vi "saveData.vi"(1 "display write dialog?":bool, 2 "append to file?":bool, 3 "Block Timing":T1) -> (0 "error out":errorcluster)   [LabVIEW 2013]
uses:
  Controls/blockTiming.ctl
  Globals/measurementGlobal.vi
panel:
  out "File Status":string="File not appended"
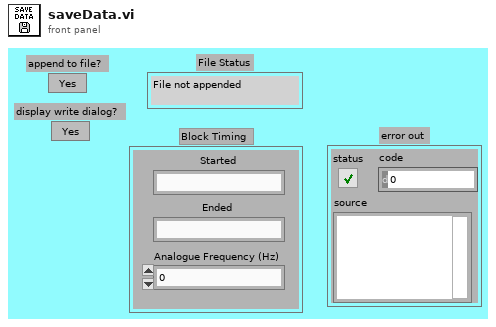
[diagram p1: front panel]
types:
  T1 = typedef "blockTiming.ctl" = cluster{"Started":string, "Ended":string, "Analogue Frequency (Hz)":dbl}
  T2 = typedef "chanType.ctl" = enum16{"Default", "Clock", "Pressure Scanner"}
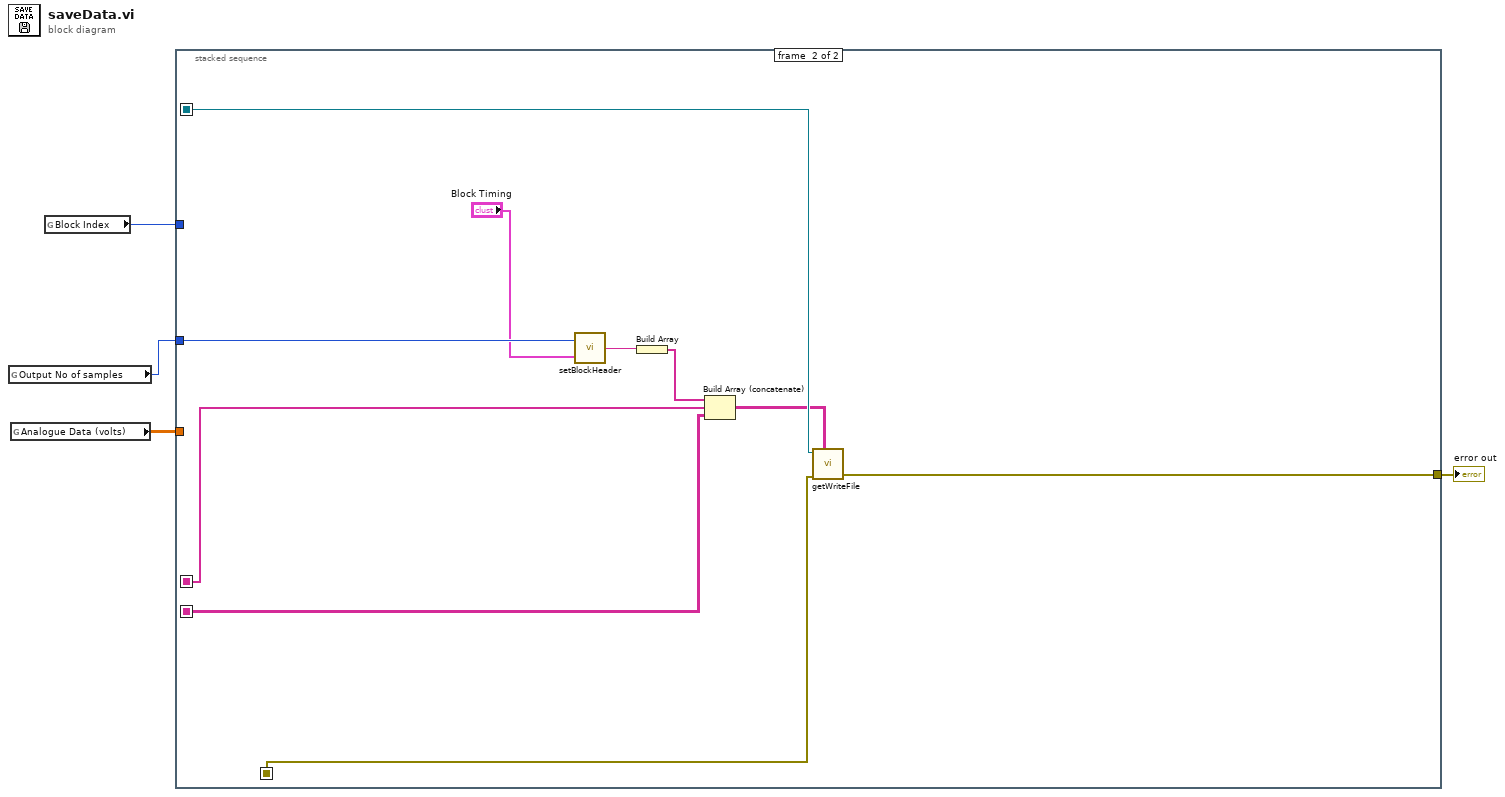
[diagram p0: block diagram]
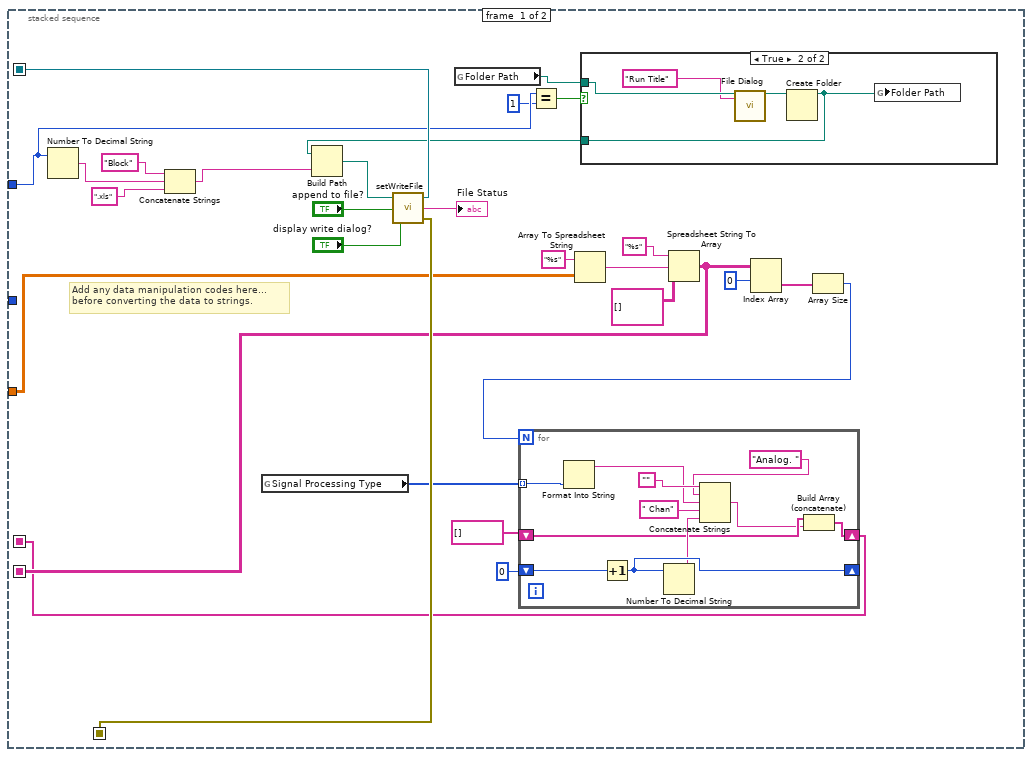
[diagram p2: hidden frame]
diagram:
  n1 = global read "measurementGlobal.vi" "Output No of samples"() -> (w3:i32)
  n2 = global read "measurementGlobal.vi" "Analogue Data (volts)"() -> (w4:dbl[][])
  n3 = global read "measurementGlobal.vi" "Block Index"() -> (w1:i32)
  n4 = stacked-sequence {
    seq-local: [w29 _] -> [_ w52]
    seq-local: [w28 _] -> [_ w51]
    seq-local: [w16 _] -> [_ w55]
    seq-local: [w15 _] -> [_ w56]
    tunnel: w4 -> [w24 _]
    tunnel: w3 -> [_ w58]
    tunnel: [_ w49] -> w2
    tunnel: w1 -> [w9 _]
    frame #0 {
      # "Add any data manipulation codes here... \nbefore converting the data to strings."
      n5 = Number To Decimal String(number=w9) -> (decimal integer string=w13:string)  [unwired: 1 in]
      n6 = Concatenate Strings("Block", w13, ".xls") -> (w11:string)
      n7 = global read "measurementGlobal.vi" "Signal Processing Type"() -> (w10:T2[])
      n8 = global read "measurementGlobal.vi" "Folder Path"() -> (w6:path)
      n9 = Equal?(x=w9, y=1) -> (x = y?=w7:bool)
      n10 = Array To Spreadsheet String(array=w24, 3:"%s" ("format string")) -> (spreadsheet string=w20:string)  [unwired: 1 in]
      n11 = case shown="True" w7 {
        tunnel: w6 -> [w33 w36]
        tunnel: [w33 w34] -> w5
        frame False {
        }
        frame True {
          n12 = call "File Dialog"("start path"=w36, "prompt"="Run Title") -> ("selected path"=w37:path)  [unwired: 10 in, 3 out]
          n13 = Create Folder(path (use dialog)=w37) -> (created path=w34:path)  [unwired: 2 in, 2 out]
          n14 = global write "measurementGlobal.vi" "Folder Path"(w34) -> ()
        }
      }
      n15 = Build Path(base path=w5, name or relative path=w11) -> (appended path=w32:path)
      n16 = call "setWriteFile.vi"("display write dialog?"="display write dialog?", "append to file?"="append to file?", "file path"=w32) -> ("error out"=w28:errorcluster, "Status"=→"File Status":string, "File Refnum"=w29:refnum<file>)
      n17 = Spreadsheet String To Array(format string="%s", spreadsheet string=w20, array type (2D Dbl)=string[][] []) -> (array=w16:string[][])  [unwired: 1 in]
      n18 = Index Array(array=w16, index (row)=0) -> (element=w22:string[])  [unwired: 1 in]
      n19 = Array Size(array=w22) -> (size(s)=w21:i32)
      n20 = for {
        N: w21 -> [_]
        shift-right: [w47] -> _
        shift-left: 0 -> [w48]
        shift-right: [w42] -> w15
        shift-left: string[] [] -> [w44]
        tunnel: w10 -> [w39] mode=indexing
        n21 = Format Into String(w39) -> (resulting string=w38:string)  [unwired: 3 in, 1 out]
        n22 = Increment(x=w48) -> (x+1=w47:i32)
        n23 = Number To Decimal String(number=w47) -> (decimal integer string=w45:string)  [unwired: 1 in]
        n24 = Concatenate Strings("", "Analog. " ("string"), w38, " Chan" ("string"), w45) -> (w43:string)
        n25 = Build Array (concatenate)(w44, w43) -> (w42:string[])
      }
    }
    frame #1 {
      n26 = call "setBlockHeader.vi"("Block Timing"="Block Timing", "No of Analog. Samples"=w58) -> ("Output String"=w54:string)
      n27 = Build Array(w54) -> (w53:string[])
      n28 = Build Array (concatenate)(w53, w56, w55) -> (w50:string[][])
      n29 = call "getWriteFile.vi"("refnum in"=w52, "error in"=w51, "Data"=w50) -> ("error out"=w49:errorcluster)  [unwired: 2 in, 2 out]
    }
  }
  "error out" <- w2
